vi "InitGlobalLogQueueAndEvent.vi"(8 "error in (no error)":errorcluster, 11 "TestCase in":refnum<class "testcase-CSMGlobalLog.lvclass">) -> (0 "error out":errorcluster, 1 "Global Log Event":refnum<user-event>, 2 "Global Log Queue":refnum<queue>, 3 "TestCase out":refnum<class "testcase-CSMGlobalLog.lvclass">)   [LabVIEW 2017, in "testcase-CSMGlobalLog.lvclass"]
uses:
  testcase-CSMGlobalLog.lvclass
  src/user.lib/_NEVSTOP/Communicable State Machine(CSM)/_Support/Typedef/_CSM_GlobalLog_MSG.ctl
  src/user.lib/_NEVSTOP/Communicable State Machine(CSM)/_Support/Typedef/_CSM_Response Source Message.ctl
  src/user.lib/_NEVSTOP/Communicable State Machine(CSM)/_Support/Typedef/_CSM_GlobalLog_MSG_TYPE.ctl
  testcase-CSMGlobalLog.lvclass/testcase-CSMGlobalLog.ctl
  src/user.lib/_NEVSTOP/Communicable State Machine(CSM)/Communicable State Machine.lvlib
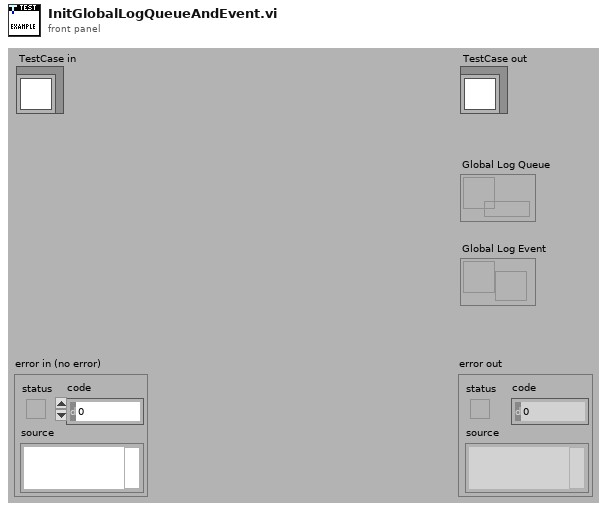
[diagram p1: front panel]
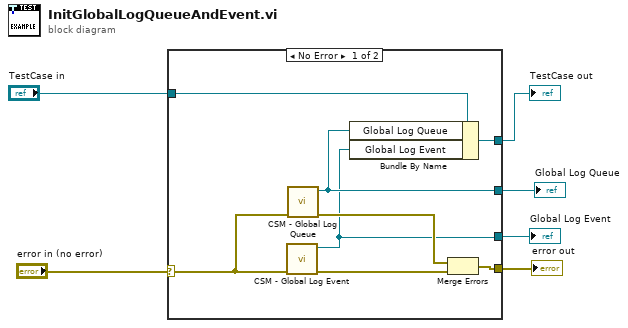
[diagram p0: block diagram]
diagram:
  n1 = case shown="No Error" "error in (no error)" {
    selector: "error in (no error)" -> [w10 w16]
    tunnel: [w12 _] -> w2
    tunnel: [w9 w16] -> w6
    tunnel: "TestCase in" -> [w13 w15]
    tunnel: [w11 w15] -> w3
    tunnel: [w7 _] -> w1
    frame No Error {
      n2 = call "CSM - Global Log Event.vi"("Error In"=w10) -> ("error out"=w8:errorcluster, "Global Log Event"=w7:refnum<user-event>)  [unwired: 9 in]
      n3 = call "CSM - Global Log Queue.vi"("Error In"=w10) -> ("error out"=w14:errorcluster, "Global Log Queue"=w12:refnum<queue>)  [unwired: 9 in]
      n4 = Bundle By Name(cluster=w13, "Global Log Queue"=w12, "Global Log Event"=w7) -> (w11:refnum<class "testcase-CSMGlobalLog.lvclass">)
      n5 = Merge Errors(w14, w8) -> (w9:errorcluster)
    }
    frame Error {
    }
  }
  "error out" <- w6
  "TestCase out" <- w3
  "Global Log Queue" <- w2
  "Global Log Event" <- w1
